vi "Get Status List From Term.vi"(5 "CSM CaseRef":refnum<vi>, 6 "need Symbol?":bool, 9 "Term Refnum":refnum<vi>) -> (3 "Array":cluster{"Status":string, "InState":string}[](array[cluster]))   [LabVIEW 2017, in "CSM-Helper.lvclass"]
uses:
  CSM-Helper.lvclass
  _Shared/Trim Single-line Text.vi
  Utility/_Support/Terminals.llb/csmHelper-Terminals.lvlib
  Utility/_Support/Relationship.llb/csmHelper-Relationship.lvlib
  _Shared/CSM Shared.lvlib
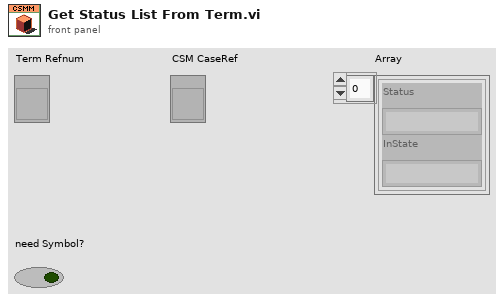
[diagram p1: front panel]
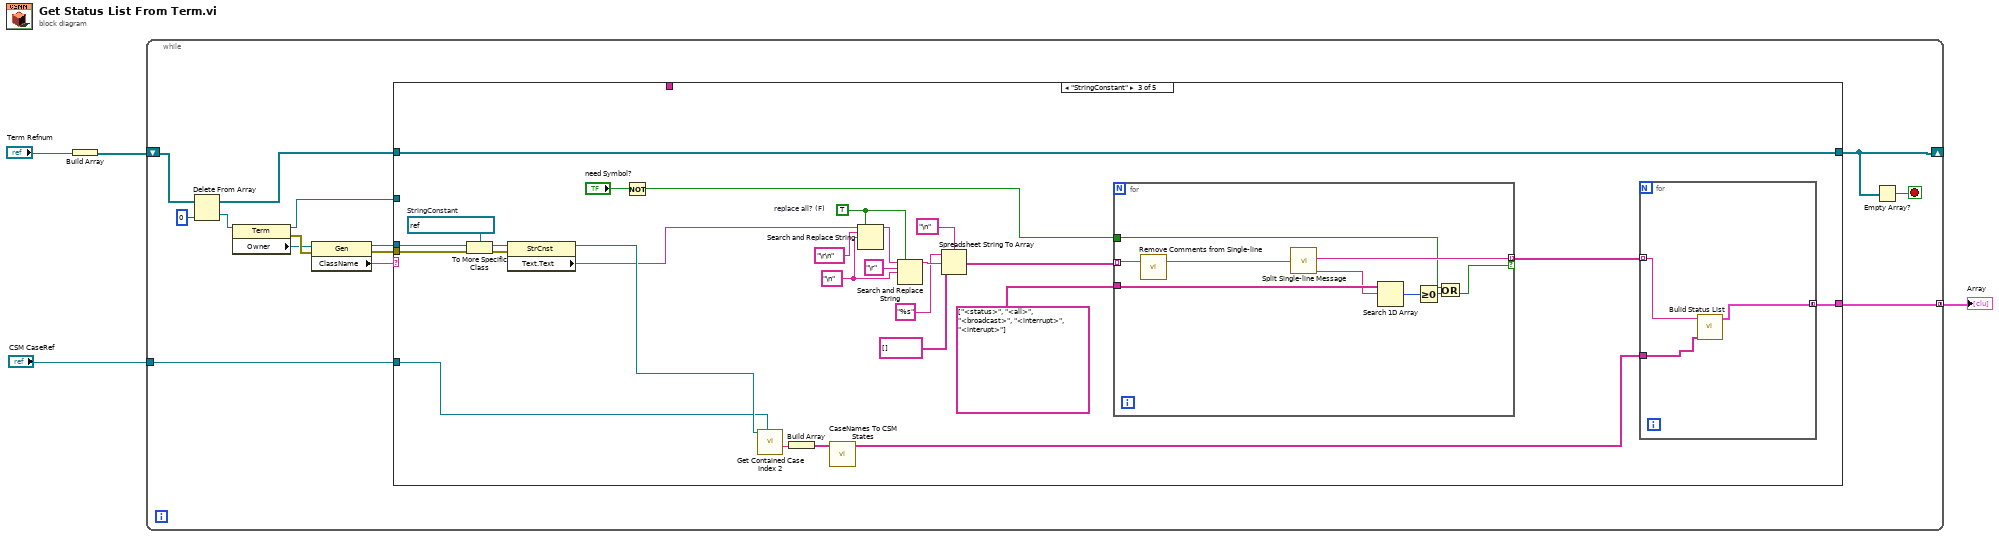
[diagram p0: block diagram]
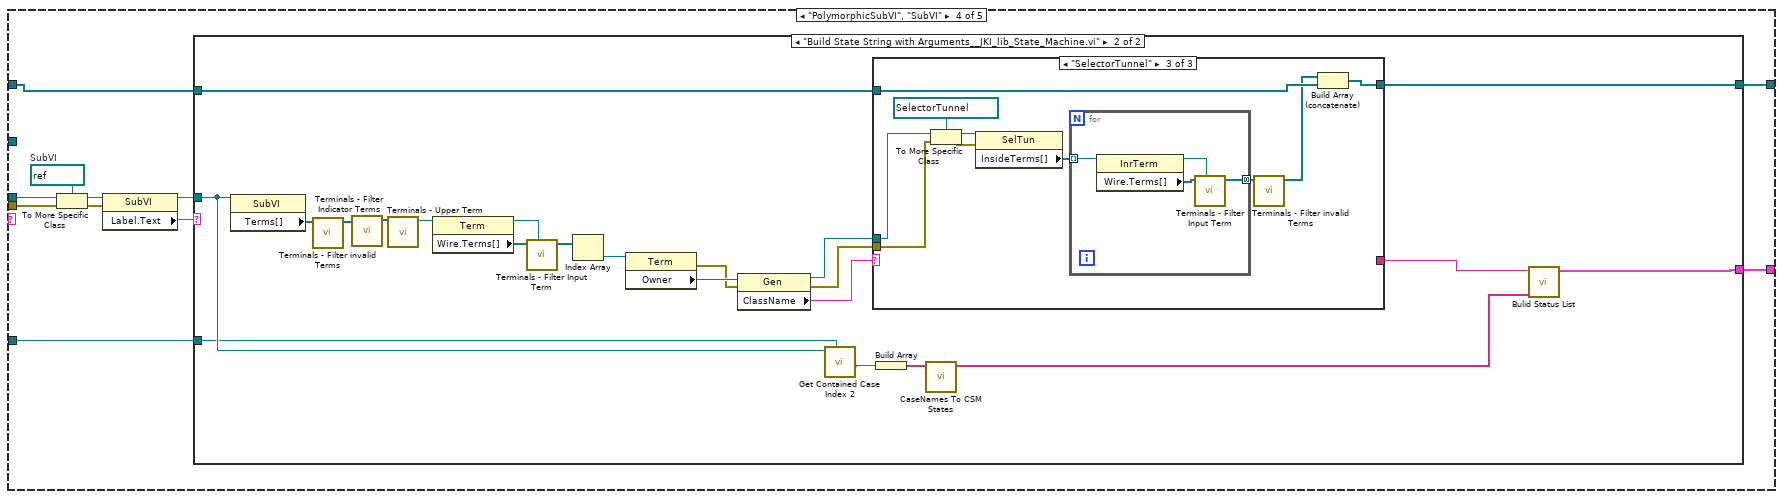
[diagram p4: hidden frame]
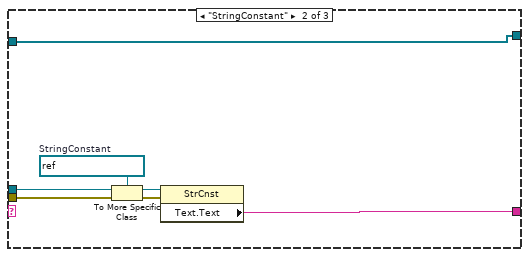
[diagram p7: hidden frame]
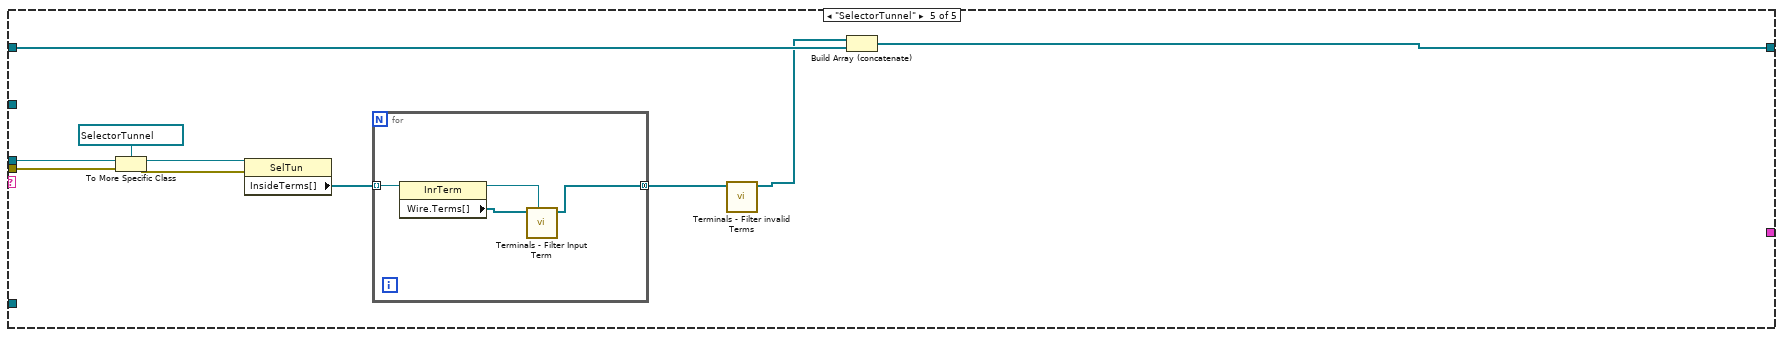
[diagram p8: hidden frame]
diagram:
  n1 = Build Array("Term Refnum") -> (w1:refnum<vi>[])
  n2 = while {
    tunnel: "CSM CaseRef" -> [w18]
    tunnel: [w17] -> w3 mode=concatenating
    shift-right: [w7] -> _
    shift-left: w1 -> [w11]
    stop <- w6 stop-if-true
    n3 = Delete From Array(array=w11, index=0) -> (deleted portion=w9:refnum<vi>, array with subset deleted=w8:refnum<vi>[])  [unwired: 1 in]
    n4 = property class="Term"(reference=w9) -> (reference out=w5:refnum<vi>, error out=w13:errorcluster, "Owner"=w12:refnum<vi>)  [unwired: 1 in]
    n5 = property class="Gen"(reference=w12, error in=w13) -> (reference out=w15:refnum<vi>, error out=w16:errorcluster, "ClassName"=w14:string)
    n6 = case shown="\"StringConstant\"" w14 {
      selector: w14 -> [w19 _ _ _ _]
      tunnel: w15 -> [_ _ w48 w71 w123]
      tunnel: w16 -> [_ _ w46 w69 w124]
      tunnel: [_ _ w42 w64 _] -> w17
      tunnel: w18 -> [_ _ w34 w63 _]
      tunnel: w8 -> [w20 w21 w36 w61 w126]
      tunnel: [w20 w21 w36 w62 w120] -> w7
      tunnel: w5 -> [_ _ _ _ _]
      tunnel: [w19 _ _ _ _] -> _
      frame "False", Default {
      }
      frame "" {
      }
      frame "StringConstant" {
        w26 = TRUE  # replace all? (F)
        w27 = "\n" ("delimiter (Tab)")
        w44 = refnum<vi> refnum  # StringConstant
        n7 = To More Specific Class(target class=w44, reference=w48, error in=w46) -> (specific class reference=w47:refnum<vi>, error out=w45:errorcluster)
        n8 = property class="StrCnst"(reference=w47, error in=w45) -> (reference out=w35:refnum<vi>, "Text.Text"=w22:string)  [unwired: 1 out]
        n9 = Not(x="need Symbol?") -> (.not. x?=w37:bool)
        n10 = call "Get Contained Case Index 2.vi"("Ref Case"=w34, "StringConstant in"=w35) -> ("FrameName"=w33:string)  [unwired: 6 in, 3 out]
        n11 = Build Array(w33) -> (w41:string[])
        n12 = call "CaseNames To CSM States.vi"("Array in"=w41) -> ("Array out"=w40:string[])  [unwired: 10 in]
        n13 = Search and Replace String(replace all?=w26, input string=w22, search string="\r\n" ("delimiter (Tab)"), replace string=w27) -> (result string=w28:string)  [unwired: 4 in, 3 out]
        n14 = Search and Replace String(replace all?=w26, input string=w28, search string="\r" ("delimiter (Tab)"), replace string=w27) -> (result string=w31:string)  [unwired: 4 in, 3 out]
        n15 = Spreadsheet String To Array(delimiter (Tab)="\n", format string="%s", spreadsheet string=w31, array type (2D Dbl)=string[] [] ("Array of Strings")) -> (array=w23:string[])
        n16 = for {
          tunnel: [w58] -> w43 mode=indexing if=w53
          tunnel: w23 -> [w59] mode=indexing
          tunnel: string[] ["<status>", "<all>", "<broadcast>", "<interrupt>", "<interupt>"] -> [w57]
          tunnel: w37 -> [w52]
          n17 = call "Remove Comments from Single-line.vi"("single-line text"=w59) -> ("single-line text without comments"=w60:string)  [unwired: 2 in]
          n18 = call "Split Single-line Message.vi"("single-line text"=w60) -> ("state"=w58:string, "source/target"=w56:string)  [unwired: 6 in, 2 out]
          n19 = Search 1D Array(1D array=w57, element=w56) -> (index of element=w55:i32)  [unwired: 1 in]
          n20 = Greater Or Equal To 0?(x=w55) -> (x >= 0?=w54:bool)
          n21 = Or(x=w52, y=w54) -> (x .or. y?=w53:bool)
        }
        n22 = for {
          tunnel: w43 -> [w50] mode=indexing
          tunnel: [w49] -> w42 mode=concatenating
          tunnel: w40 -> [w51]
          n23 = call "Bulid Status List.vi"("Array in"=w51, "Text.Text"=w50) -> ("Array"=w49:cluster{"Status":string, "InState":string}[])  [unwired: 9 in]
        }
      }
      frame "PolymorphicSubVI", "SubVI" {
        w67 = refnum<vi> refnum  # SubVI
        n24 = To More Specific Class(target class=w67, reference=w71, error in=w69) -> (specific class reference=w70:refnum<vi>, error out=w68:errorcluster)
        n25 = property class="SubVI"(reference=w70, error in=w68) -> (reference out=w65:refnum<vi>, "Label.Text"=w66:string)  [unwired: 1 out]
        n26 = case shown="\"Build State String with Arguments__JKI_lib_State_Machine.vi\"" w66 {
          tunnel: w65 -> [_ w78]
          tunnel: [_ w85] -> w64
          tunnel: w63 -> [_ w77]
          tunnel: w61 -> [w72 w76]
          tunnel: [w72 w75] -> w62
          frame Default {
          }
          frame "Build State String with Arguments__JKI_lib_State_Machine.vi" {
            n27 = property class="SubVI"(reference=w78) -> ("Terms[]"=w94:refnum<vi>[])  [unwired: 1 in, 2 out]
            n28 = call "Terminals - Filter invalid Terms.vi"("Terms[]"=w94) -> ("Terms[] out"=w86:refnum<vi>[])  [unwired: 10 in]
            n29 = call "Terminals - Filter Indicator Terms.vi"("Terms[]"=w86) -> ("Terms[] out"=w81:refnum<vi>[])  [unwired: 10 in]
            n30 = call "Terminals - Upper Term.vi"("Terms[]"=w81) -> ("Terms[] out"=w90:refnum<vi>)  [unwired: 10 in]
            n31 = property class="Term"(reference=w90) -> (reference out=w83:refnum<vi>, "Wire.Terms[]"=w84:refnum<vi>[])  [unwired: 1 in, 1 out]
            n32 = call "Terminals - Filter Input Term.vi"("InnerTerminal in"=w83, "Wire.Terms[] in"=w84) -> ("Wire.Terms[] out"=w82:refnum<vi>[])  [unwired: 9 in]
            n33 = Index Array(array=w82) -> (element=w93:refnum<vi>)  [unwired: 1 in]
            n34 = property class="Term"(reference=w93) -> (error out=w91:errorcluster, "Owner"=w92:refnum<vi>)  [unwired: 1 in, 1 out]
            n35 = property class="Gen"(reference=w92, error in=w91) -> (reference out=w87:refnum<vi>, error out=w88:errorcluster, "ClassName"=w89:string)
            n36 = call "Get Contained Case Index 2.vi"("Ref Case"=w77, "StringConstant in"=w78) -> ("FrameName"=w79:string)  [unwired: 6 in, 3 out]
            n37 = case shown="\"SelectorTunnel\"" w89 {
              tunnel: w87 -> [_ w102 w106]
              tunnel: w88 -> [_ w100 w105]
              tunnel: [_ w97 _] -> w74
              tunnel: w76 -> [w95 w96 w107]
              tunnel: [w95 w96 w104] -> w75
              frame Default {
              }
              frame "StringConstant" {
                w98 = refnum<vi> refnum  # StringConstant
                n38 = To More Specific Class(target class=w98, reference=w102, error in=w100) -> (specific class reference=w101:refnum<vi>, error out=w99:errorcluster)
                n39 = property class="StrCnst"(reference=w101, error in=w99) -> ("Text.Text"=w97:string)  [unwired: 2 out]
              }
              frame "SelectorTunnel" {
                n40 = To More Specific Class(target class=refnum<vi> refnum ("reference out"), reference=w106, error in=w105) -> (specific class reference=w112:refnum<vi>, error out=w111:errorcluster)
                n41 = property class="SelTun"(reference=w112, error in=w111) -> ("InsideTerms[]"=w110:refnum<vi>[])  [unwired: 2 out]
                n42 = for {
                  tunnel: w110 -> [w116] mode=indexing
                  tunnel: [w113] -> w109 mode=concatenating
                  n43 = property class="InrTerm"(reference=w116) -> (reference out=w114:refnum<vi>, "Wire.Terms[]"=w115:refnum<vi>[])  [unwired: 1 in, 1 out]
                  n44 = call "Terminals - Filter Input Term.vi"("InnerTerminal in"=w114, "Wire.Terms[] in"=w115) -> ("Wire.Terms[] out"=w113:refnum<vi>[])  [unwired: 9 in]
                }
                n45 = call "Terminals - Filter invalid Terms.vi"("Terms[]"=w109) -> ("Terms[] out"=w103:refnum<vi>[])  [unwired: 10 in]
                n46 = Build Array (concatenate)(w103, w107) -> (w104:refnum<vi>[])
              }
            }
            n47 = Build Array(w79) -> (w80:string[])
            n48 = call "CaseNames To CSM States.vi"("Array in"=w80) -> ("Array out"=w73:string[])  [unwired: 10 in]
            n49 = call "Bulid Status List.vi"("Array in"=w73, "Text.Text"=w74) -> ("Array"=w85:cluster{"Status":string, "InState":string}[])  [unwired: 9 in]
          }
        }
      }
      frame "SelectorTunnel" {
        n50 = To More Specific Class(target class=refnum<vi> refnum ("reference out"), reference=w123, error in=w124) -> (specific class reference=w122:refnum<vi>, error out=w121:errorcluster)
        n51 = property class="SelTun"(reference=w122, error in=w121) -> ("InsideTerms[]"=w119:refnum<vi>[])  [unwired: 2 out]
        n52 = for {
          tunnel: w119 -> [w130] mode=indexing
          tunnel: [w127] -> w118 mode=concatenating
          n53 = property class="InrTerm"(reference=w130) -> (reference out=w128:refnum<vi>, "Wire.Terms[]"=w129:refnum<vi>[])  [unwired: 1 in, 1 out]
          n54 = call "Terminals - Filter Input Term.vi"("InnerTerminal in"=w128, "Wire.Terms[] in"=w129) -> ("Wire.Terms[] out"=w127:refnum<vi>[])  [unwired: 9 in]
        }
        n55 = call "Terminals - Filter invalid Terms.vi"("Terms[]"=w118) -> ("Terms[] out"=w117:refnum<vi>[])  [unwired: 10 in]
        n56 = Build Array (concatenate)(w117, w126) -> (w120:refnum<vi>[])
      }
    }
    n57 = Empty Array?(array=w7) -> (empty?=w6:bool)
  }
  "Array" <- w3
